vi "Initialization.vi"(8 "error in (no error)":errorcluster, 11 "DAQmxTaksContainer_Emulate in":refnum<class "DAQmxTaksContainer_Emulate.lvclass">) -> (0 "error out":errorcluster, 3 "DAQmxTaksContainer_Emulate out":refnum<class "DAQmxTaksContainer_Emulate.lvclass">)   [LabVIEW 2020, in "DAQmxTaksContainer_Emulate.lvclass"]
uses:
  DAQmxTaksContainer_Emulate.lvclass
  C:/dev/TRANCON/Classes/GeneralFunctionality/GeneralFunctionality.lvclass
  C:/dev/TRANCON/Classes/DAQmxTasks/DAQmxTaskContainer_General/DAQmxTaksContainer_General.lvclass
  GeneralFunctionality/GeneralFunctionality.lvclass/GeneralFunctionality.ctl
  Config/Config.lvclass/Config.ctl
  dependecies/ControlsVIs/Clusters-def/list-of-keys-DAQmx-tasks.ctl
  DAQmxTaskDInput_Emulate/DAQmxTaskDInput_Emulate.lvclass
  C:/dev/TRANCON/Classes/DAQmxTasks/DAQmxTask.lvclass
  DAQmxTaskAICurrent_Emulate/DAQmxTaskAICurrent_Emulate.lvclass
  C:/dev/TRANCON/Classes/DAQmxTasks/DAQmxTaskAICurrent_General/DAQmxTaskAICurrent_General.lvclass
  DAQmxTaskContainer_General/DAQmxTaksContainer_General.lvclass/DAQmxTaksContainer_General.ctl
  DAQmxTaskAICurrent_General/DAQmxTaskAICurrent_General.lvclass/DAQmxTaskAICurrent_General.ctl
  DAQmxTask.lvclass/DAQmxTask.ctl
  DAQmxTaskAITension_Emulate/DAQmxTaskAIVoltage_Emulate.lvclass
  C:/dev/TRANCON/Classes/DAQmxTasks/DAQmxTaskAITension_General/DAQmxTaskAIVoltage_General.lvclass
  DAQmxTaskAITension_General/DAQmxTaskAIVoltage_General.lvclass/DAQmxTaskAIVoltage_General.ctl
  DAQmxTaskDOutput_Emulate/DAQmxTaskDOutput_Emulate.lvclass
  DAQmxTaskCounterDigital_Emulate/DAQmxTaskCounterDigital_Emulate.lvclass
  Config/Config.lvclass
  DAQmxTask.lvclass
  DAQmxTaskContainer_General/DAQmxTaksContainer_General.lvclass
  GeneralFunctionality/GeneralFunctionality.lvclass
  DAQmxTaskAICurrent_General/DAQmxTaskAICurrent_General.lvclass
  DAQmxTaskAITension_General/DAQmxTaskAIVoltage_General.lvclass
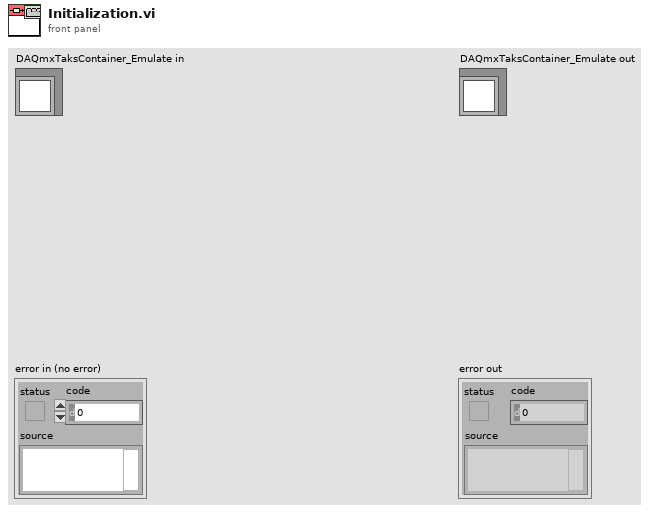
[diagram p1: front panel]
types:
  T1 = typedef "DAQmxTaksContainer_General.lvclass/list-of-keys-DAQmx-tasks.ctl" = string
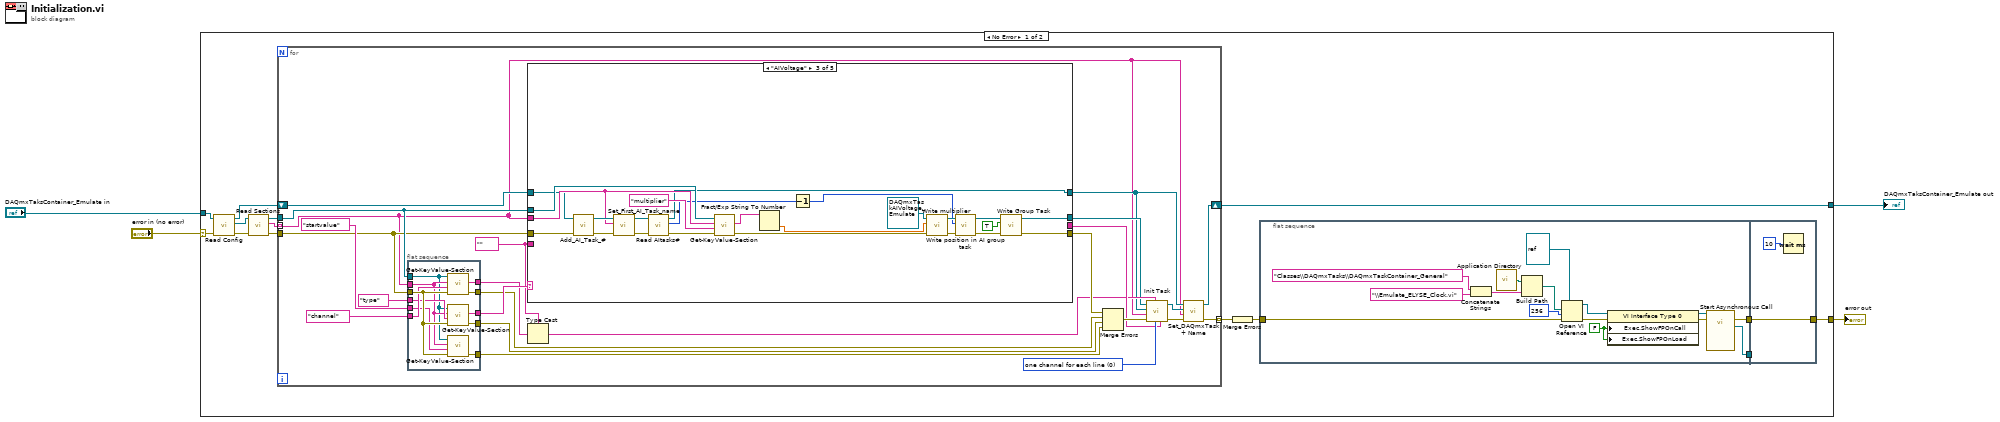
[diagram p0: block diagram]
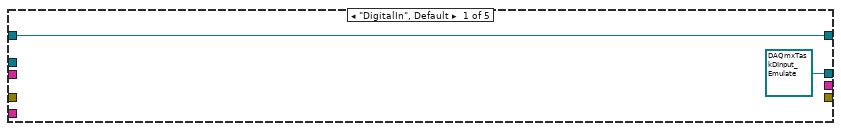
[diagram p2: hidden frame]
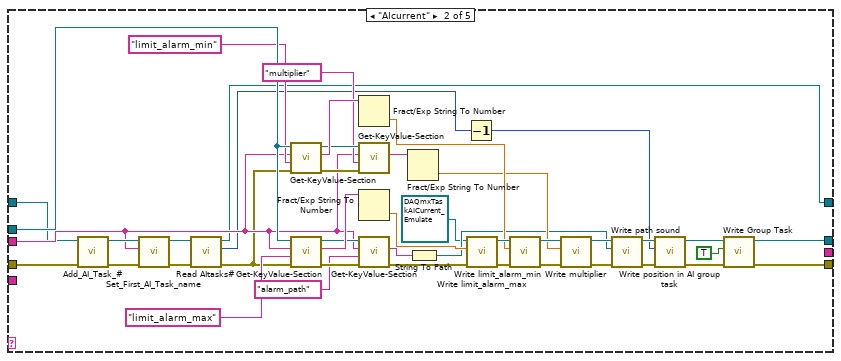
[diagram p3: hidden frame]
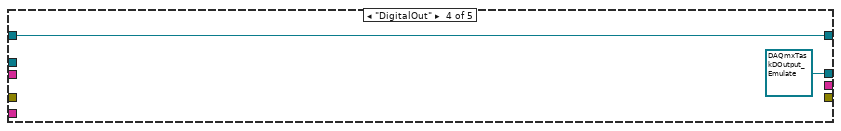
[diagram p4: hidden frame]
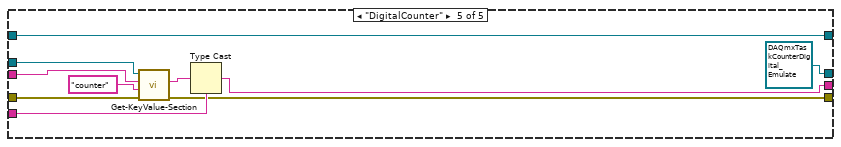
[diagram p5: hidden frame]
diagram:
  n1 = case shown="No Error" "error in (no error)" {
    selector: "error in (no error)" -> [w14 w152]
    tunnel: [w8 w152] -> w2
    tunnel: [w7 w153] -> w1
    tunnel: "DAQmxTaksContainer_Emulate in" -> [w6 w153]
    frame No Error {
      n2 = call "Read Config.vi"("error in (no error)"=w14, "GeneralFunctionality en entrée"=w6) -> ("error out"=w13:errorcluster, "Config.lvclass"=w12:refnum<class "Config.lvclass">, "GeneralFunctionality en sortie"=w5:refnum<class "DAQmxTaksContainer_Emulate.lvclass">)  [unwired: 7 in]
      n3 = call "Read Sections.vi"("error in (no error)"=w13, "Config in"=w12) -> ("error out"=w17:errorcluster, "Sections"=w16:string[], "Config out"=w18:refnum<class "Config.lvclass">)  [unwired: 7 in]
      n4 = for {
        tunnel: w16 -> [w36] mode=indexing
        tunnel: w17 -> [w47]
        tunnel: w18 -> [w54]
        tunnel: [w40] -> w15 mode=indexing
        shift-right: [w38] -> w7
        shift-left: w5 -> [w42]
        w50 = 0 items=["one channel for each line", "one channel for all lines"] ("line grouping")
        w48 = tag "" ("physical channels")
        n5 = flat-sequence {
          tunnel: w47 -> [w70]
          tunnel: T1 "channel" ("Key") -> [w69]
          tunnel: T1 "type" ("Key") -> [w68]
          tunnel: T1 "startvalue" ("Key") -> [w67]
          tunnel: [w66] -> w56
          tunnel: [w65] -> w55
          tunnel: w36 -> [w64]
          tunnel: w54 -> [w63]
          tunnel: [w62] -> w53
          tunnel: [w61] -> w52
          tunnel: [w60] -> w51
          frame #0 {
            n6 = call-dynamic "Get-KeyValue-Section.vi"("error in (no error)"=w70, "Key"=w69, "Section"=w64, "Config in"=w63) -> ("error out"=w62:errorcluster, "Value"=w65:string)  [unwired: 5 in, 1 out]
            n7 = call-dynamic "Get-KeyValue-Section.vi"("error in (no error)"=w70, "Key"=w68, "Section"=w64, "Config in"=w63) -> ("error out"=w61:errorcluster, "Value"=w66:string)  [unwired: 5 in, 1 out]
            n8 = call-dynamic "Get-KeyValue-Section.vi"("error in (no error)"=w70, "Key"=w67, "Section"=w64, "Config in"=w63) -> ("error out"=w60:errorcluster)  [unwired: 5 in, 2 out]
          }
        }
        n9 = case shown="\"AIVoltage\"" w56 {
          tunnel: w54 -> [_ w106 w137 _ w147]
          tunnel: [refnum<class "DAQmxTaskDInput_Emulate.lvclass"> refnum ("DAQmxTaskDInput_Emulate.lvclass") w79 w122 refnum<class "DAQmxTaskDOutput_Emulate.lvclass"> refnum ("DAQmxTaskDOutput_Emulate.lvclass") refnum<class "DAQmxTaskCounterDigital_Emulate.lvclass"> refnum ("DAQmxTaskCounterDigital_Emulate.lvclass")] -> w43
          tunnel: w48 -> [_ _ _ _ w151]
          tunnel: [_ _ _ _ w149] -> w45
          tunnel: w36 -> [_ w87 w130 _ w148]
          tunnel: w47 -> [_ w90 w131 _ w145]
          tunnel: [_ w80 w123 _ w144] -> w46
          tunnel: [w71 w82 w125 w140 w142] -> w39
          tunnel: w42 -> [w71 w86 w129 w140 w142]
          frame "DigitalIn", Default {
          }
          frame "AIcurrent" {
            n10 = call "Add_AI_Task_#.vi"("error in (no error)"=w90, "DAQmxTaksContainer_General in"=w86) -> ("error out"=w89:errorcluster, "DAQmxTaksContainer_General out"=w88:refnum<class "DAQmxTaksContainer_Emulate.lvclass">)  [unwired: 8 in]
            n11 = call "Set_First_AI_Task_name.vi"("error in (no error)"=w89, "Name"=w87, "DAQmxTaksContainer_General in"=w88) -> ("error out"=w85:errorcluster, "DAQmxTaksContainer_General out"=w83:refnum<class "DAQmxTaksContainer_Emulate.lvclass">)  [unwired: 7 in]
            n12 = call "Read AItasks#.vi"("error in (no error)"=w85, "DAQmxTaksContainer_General in"=w83) -> ("error out"=w84:errorcluster, "AItasks#"=w81:i32, "DAQmxTaksContainer_General out"=w82:refnum<class "DAQmxTaksContainer_Emulate.lvclass">)  [unwired: 7 in]
            n13 = call-dynamic "Get-KeyValue-Section.vi"("error in (no error)"=w84, "Key"="limit_alarm_min", "Section"=w87, "Config in"=w106) -> ("error out"=w101:errorcluster, "Value"=w104:string, "Config out"=w102:refnum<class "Config.lvclass">)  [unwired: 5 in]
            n14 = call-dynamic "Get-KeyValue-Section.vi"("error in (no error)"=w84, "Key"="limit_alarm_max", "Section"=w87, "Config in"=w106) -> ("error out"=w97:errorcluster, "Value"=w108:string, "Config out"=w95:refnum<class "Config.lvclass">)  [unwired: 5 in]
            n15 = Fract/Exp String To Number(string=w104) -> (number=w103:dbl)  [unwired: 3 in, 1 out]
            n16 = call-dynamic "Get-KeyValue-Section.vi"("error in (no error)"=w101, "Key"="multiplier", "Section"=w87, "Config in"=w102) -> ("Value"=w99:string)  [unwired: 5 in, 2 out]
            n17 = Fract/Exp String To Number(string=w108) -> (number=w107:dbl)  [unwired: 3 in, 1 out]
            n18 = call-dynamic "Get-KeyValue-Section.vi"("error in (no error)"=w97, "Key"="alarm_path", "Section"=w87, "Config in"=w95) -> ("error out"=w96:errorcluster, "Value"=w93:string)  [unwired: 5 in, 1 out]
            n19 = Fract/Exp String To Number(string=w99) -> (number=w98:dbl)  [unwired: 3 in, 1 out]
            n20 = String To Path(string=w93) -> (path=w92:path)
            n21 = Decrement(x=w81) -> (x-1=w74:i32)
            n22 = call "Write limit_alarm_max.vi"("error in (no error)"=w96, "limit_alarm_max"=w107, "DAQmxTaskAICurrent_General in"=refnum<class "DAQmxTaskAICurrent_Emulate.lvclass"> refnum ("DAQmxTaskAICurrent_Emulate.lvclass")) -> ("error out"=w112:errorcluster, "DAQmxTaskAICurrent_General out"=w115:refnum<class "DAQmxTaskAICurrent_Emulate.lvclass">)  [unwired: 7 in]
            n23 = call "Write limit_alarm_min.vi"("error in (no error)"=w112, "limit_alarm_min"=w103, "DAQmxTaskAICurrent_General in"=w115) -> ("error out"=w111:errorcluster, "DAQmxTaskAICurrent_General out"=w114:refnum<class "DAQmxTaskAICurrent_Emulate.lvclass">)  [unwired: 7 in]
            n24 = call "Write multiplier.vi"("error in (no error)"=w111, "multiplier"=w98, "DAQmxTaskAICurrent_General in"=w114) -> ("error out"=w110:errorcluster, "DAQmxTaskAICurrent_General out"=w113:refnum<class "DAQmxTaskAICurrent_Emulate.lvclass">)  [unwired: 7 in]
            n25 = call "Write path sound.vi"("error in (no error)"=w110, "path sound"=w92, "DAQmxTaskAICurrent_General in"=w113) -> ("error out"=w73:errorcluster, "DAQmxTaskAICurrent_General out"=w75:refnum<class "DAQmxTaskAICurrent_Emulate.lvclass">)  [unwired: 7 in]
            n26 = call "Write position in AI group task.vi"("error in (no error)"=w73, "position in AI group task"=w74, "DAQmxTask in"=w75) -> ("error out"=w77:errorcluster, "DAQmxTask out"=w76:refnum<class "DAQmxTaskAICurrent_Emulate.lvclass">)  [unwired: 7 in]
            n27 = call "Write Group Task.vi"("error in (no error)"=w77, "Group Task"=TRUE, "DAQmxTask in"=w76) -> ("error out"=w80:errorcluster, "DAQmxTask out"=w79:refnum<class "DAQmxTaskAICurrent_Emulate.lvclass">)  [unwired: 7 in]
          }
          frame "AIVoltage" {
            n28 = call "Add_AI_Task_#.vi"("error in (no error)"=w131, "DAQmxTaksContainer_General in"=w129) -> ("error out"=w133:errorcluster, "DAQmxTaksContainer_General out"=w132:refnum<class "DAQmxTaksContainer_Emulate.lvclass">)  [unwired: 8 in]
            n29 = call "Set_First_AI_Task_name.vi"("error in (no error)"=w133, "Name"=w130, "DAQmxTaksContainer_General in"=w132) -> ("error out"=w128:errorcluster, "DAQmxTaksContainer_General out"=w126:refnum<class "DAQmxTaksContainer_Emulate.lvclass">)  [unwired: 7 in]
            n30 = call "Read AItasks#.vi"("error in (no error)"=w128, "DAQmxTaksContainer_General in"=w126) -> ("error out"=w127:errorcluster, "AItasks#"=w124:i32, "DAQmxTaksContainer_General out"=w125:refnum<class "DAQmxTaksContainer_Emulate.lvclass">)  [unwired: 7 in]
            n31 = call-dynamic "Get-KeyValue-Section.vi"("error in (no error)"=w127, "Key"="multiplier", "Section"=w130, "Config in"=w137) -> ("error out"=w136:errorcluster, "Value"=w138:string)  [unwired: 5 in, 1 out]
            n32 = Fract/Exp String To Number(string=w138) -> (number=w134:dbl)  [unwired: 3 in, 1 out]
            n33 = Decrement(x=w124) -> (x-1=w117:i32)
            n34 = call "Write multiplier.vi"("error in (no error)"=w136, "multiplier"=w134, "DAQmxTaskAIVoltage_General in"=refnum<class "DAQmxTaskAIVoltage_Emulate.lvclass"> refnum ("DAQmxTaskAITension_Emulate.lvclass")) -> ("error out"=w116:errorcluster, "DAQmxTaskAIVoltage_General out"=w118:refnum<class "DAQmxTaskAIVoltage_Emulate.lvclass">)  [unwired: 7 in]
            n35 = call "Write position in AI group task.vi"("error in (no error)"=w116, "position in AI group task"=w117, "DAQmxTask in"=w118) -> ("error out"=w120:errorcluster, "DAQmxTask out"=w119:refnum<class "DAQmxTaskAIVoltage_Emulate.lvclass">)  [unwired: 7 in]
            n36 = call "Write Group Task.vi"("error in (no error)"=w120, "Group Task"=TRUE, "DAQmxTask in"=w119) -> ("error out"=w123:errorcluster, "DAQmxTask out"=w122:refnum<class "DAQmxTaskAIVoltage_Emulate.lvclass">)  [unwired: 7 in]
          }
          frame "DigitalOut" {
          }
          frame "DigitalCounter" {
            n37 = call-dynamic "Get-KeyValue-Section.vi"("error in (no error)"=w145, "Key"="counter", "Section"=w148, "Config in"=w147) -> ("error out"=w144:errorcluster, "Value"=w150:string)  [unwired: 5 in, 1 out]
            n38 = Type Cast(type=w151, x=w150) -> (*(type *) &x=w149:tag)
          }
        }
        n39 = Type Cast(type=w48, x=w55) -> (*(type *) &x=w44:tag)
        n40 = Merge Errors(w46, w53, w52, w51) -> (w49:errorcluster)
        n41 = call-dynamic "Init Task.vi"("counter"=w45, "line grouping"=w50, "physical channels"=w44, "error in (no error)"=w49, "name"=w36, "DAQmxTaksContainer_General IN"=w39, "DAQmxTask in"=w43) -> ("error out"=w41:errorcluster, "DAQmxTask OUT"=w37:refnum<class "DAQmxTask.lvclass">)  [unwired: 3 in]
        n42 = call "Set_DAQmxTask + Name.vi"("error in (no error)"=w41, "Task name"=w36, "DAQmxTask.lvclass"=w37, "DAQmxTaksContainer_General in"=w39) -> ("error out"=w40:errorcluster, "DAQmxTaksContainer_General out"=w38:refnum<class "DAQmxTaksContainer_Emulate.lvclass">)  [unwired: 6 in]
      }
      n43 = Merge Errors(w15) -> (w9:errorcluster)
      n44 = flat-sequence {
        tunnel: [w33] -> w11
        tunnel: [w23] -> w10
        tunnel: w9 -> [w20]
        tunnel: w11 -> [w34]
        tunnel: w10 -> [_]
        tunnel: [w34] -> w8
        frame #0 {
          w27 = FALSE ("Execution:Show Front Panel On Call")
          n45 = Concatenate Strings("Classes\\DAQmxTasks\\DAQmxTaskContainer_General" ("chaîne"), "\\Emulate_ELYSE_Clock.vi" ("chaîne")) -> (w26:string)
          n46 = call <vilib>:"Application Directory.vi"() -> ("Application Directory"=w31:path)
          n47 = Build Path(base path=w31, name or relative path=w26) -> (appended path=w32:path)
          n48 = Open VI Reference(type specifier VI Refnum (for type only)=refnum<vi> refnum ("spécificateur de type du refnum de VI (pour type seulement)"), vi path=w32, options=256, error in (no error)=w20) -> (vi reference=w22:refnum<vi>, error out=w28:errorcluster)  [unwired: 2 in]
          n49 = property class="VI Interface Type 0"(reference=w22, error in=w28, "Exec.ShowFPOnCall"=w27, "Exec.ShowFPOnLoad"=w27) -> (reference out=w21:refnum<vi>, error out=w19:errorcluster)
          n50 = call-by-ref "Start Asynchronous Call"(reference=w21, error in=w19) -> (reference out=w23:refnum<vi>, error out=w33:errorcluster)  [unwired: 12 in]
        }
        frame #1 {
          n51 = Wait (ms)(milliseconds to wait=u32 10) -> ()  [unwired: 1 out]
        }
      }
    }
    frame Error {
    }
  }
  "error out" <- w2
  "DAQmxTaksContainer_Emulate out" <- w1
